vi "Set Shooter Wheel.vi"(2 "Reverse":bool, 3 "Motor Speed":dbl) -> ()   [LabVIEW 2013]
uses:
  Robot Global Data.vi
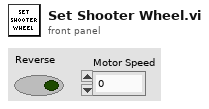
[diagram p1: front panel]
types:
  T1 = typedef "WPI_MotorControlDeviceRef.ctl" = cluster{"DeviceStatus":errorcluster, "Type":enum16{"PWM", "CAN"}, "PWM":cluster{"Digital Module":T2, "PWM Channel":T3, "DeadBand":T4}, "CAN":cluster{"Device Number":u8, "Control Mode":T5, "Semaphore":T6, "Max Vout":dbl}, "Invert":bool, "TransformRef":T7, "InvTransformRef":T7}
  T2 = typedef "FPGA_TypedefDigitalModule.ctl" = enum16{"Digital Module 1", "Digital Module 2"}
  T3 = typedef "FPGA_DIOPWMChannel.ctl" = enum8{"PWM 1", "PWM 2", "PWM 3", "PWM 4", "PWM 5", "PWM 6", "PWM 7", "PWM 8", "PWM 9", "PWM 10", "Invalid"}
  T4 = typedef "WPI_PWMDeadband.ctl" = cluster{"Name":string, "maxPositivePwm":i32, "minPositivePwm":i32, "centerPwm":i32, "maxNegativePwm":i32, "minNegativePwm":i32, "angularRange":u16}
  T5 = typedef "WPI_CANJaguar_ControlMode.ctl" = enum8{"Percent VBus", "Current", "Speed", "Position", "Voltage"}
  T6 = typedef "Semaphore RefNum" = refnum<k1>
  T7 = typedef "WPI_PWMTransform_ConPane.ctl" = refnum<vi>
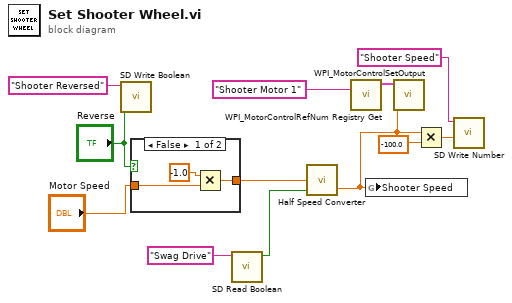
[diagram p0: block diagram]
diagram:
  n1 = call <vilib>:"SD Write Boolean.vi"("Boolean"="Reverse", "Name"="Shooter Reversed") -> ()  [unwired: 8 in, 2 out]
  n2 = case shown="False" "Reverse" {
    tunnel: [w15 w16] -> w3
    tunnel: "Motor Speed" -> [w13 w16]
    frame False {
      n3 = Multiply(x=-1.0, y=w13) -> (x*y=w15:dbl)
    }
    frame True {
    }
  }
  n4 = call <vilib>:"SD Read Boolean.vi"("Name"="Swag Drive") -> ("Boolean"=w1:bool)  [unwired: 8 in, 2 out]
  n5 = call "Half Speed Converter.vi"("Enable"=w1, "Y axis"=w3) -> ("Y axis"=w2:dbl)  [unwired: 1 in, 1 out]
  n6 = call <vilib>:"WPI_MotorControlRefNum Registry Get.vi"("refnum name"="Shooter Motor 1") -> ("MotorControlDevRef"=w11:T1)  [unwired: 9 in, 1 out]
  n7 = global write "Robot Global Data.vi" "Shooter Speed"(w2) -> ()
  n8 = call <vilib>:"WPI_MotorControlSetOutput.vi"("Output"=w2, "MotorControlDevRef"=w11) -> ()  [unwired: 7 in, 3 out]
  n9 = Multiply(x=w2, y=-100.0) -> (x*y=w7:dbl)
  n10 = call <vilib>:"SD Write Number.vi"("Numeric"=w7, "Name"="Shooter Speed") -> ()  [unwired: 8 in, 2 out]
